vi "encodeArrayVariant.vi"(5 "Cluster To Map? (T)":bool=TRUE, 7 "Compress? (T)":bool=TRUE, 8 "error in":errorcluster, 11 "Variant":variant) -> (0 "error out":errorcluster, 3 "MessagePack":u8[](array[numeric]) format="%.0x")   [LabVIEW 2015, in "MsgPack.lvlib"]
uses:
  MsgPack.lvlib
  encodeArrayInt8.vi
  encodeArrayInt16.vi
  encodeArrayInt32.vi
  encodeArrayInt64.vi
  encodeArrayUInt8.vi
  encodeArrayUInt16.vi
  encodeArrayUInt32.vi
  encodeArrayUInt64.vi
  encodeArrayFloat32.vi
  encodeArrayFloat64.vi
  encodeArrayBoolean.vi
  encodeArrayString.vi
  encodeArrayTimestamp.vi
  encodeBaseType.vi
  encodeInt8.vi
  encodeInt16.vi
  encodeInt32.vi
  encodeInt64.vi
  encodeUInt8.vi
  encodeUInt16.vi
  encodeUInt32.vi
  encodeUInt64.vi
  encodeFloat32.vi
  encodeFloat64.vi
  SubVis/encodeBooleanRaw.vi
  encodeString.vi
  encodeTimestamp.vi
  SubVis/encodeFixedInt.vi
  encodeExt.vi
  <vilib>/ErrorRing/Error Ring.xnode
  <vilib>/Utility/Data Type/NI_Data Type.lvlib
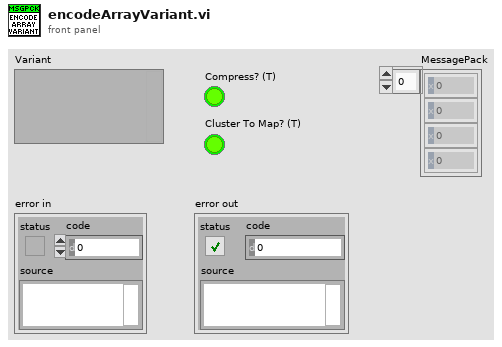
[diagram p1: front panel]
types:
  T1 = typedef "NI_Data Type.lvlib/Data Type.ctl" = enum8{"Invalid Type", "Void", "I8", "I16", "I32", "I64", "U8", "U16", "U32", "U64", "Single Float", "Double Float", "Extended Float", "Single Complex", "Double Complex", "Extended Complex", "Enum U8", "Enum U16", "Enum U32", "Enum U64", "Single Float With Unit", "Double Float With Unit", "Extended Float With Unit", "Single Complex with Unit", "Double Complex with Unit", "Extended Complex with Unit", "Boolean", "String", "Path", "Picture", "Tag", "Array", "Cluster", "Variant", "LV Variant", "Waveform", "Timestamp", "Digital Waveform", "Digital Data", "ExpressData", "Refnum", "External Data", "VI", "Poly VI", "LabVIEW Class Instance", "Fixed Point"}
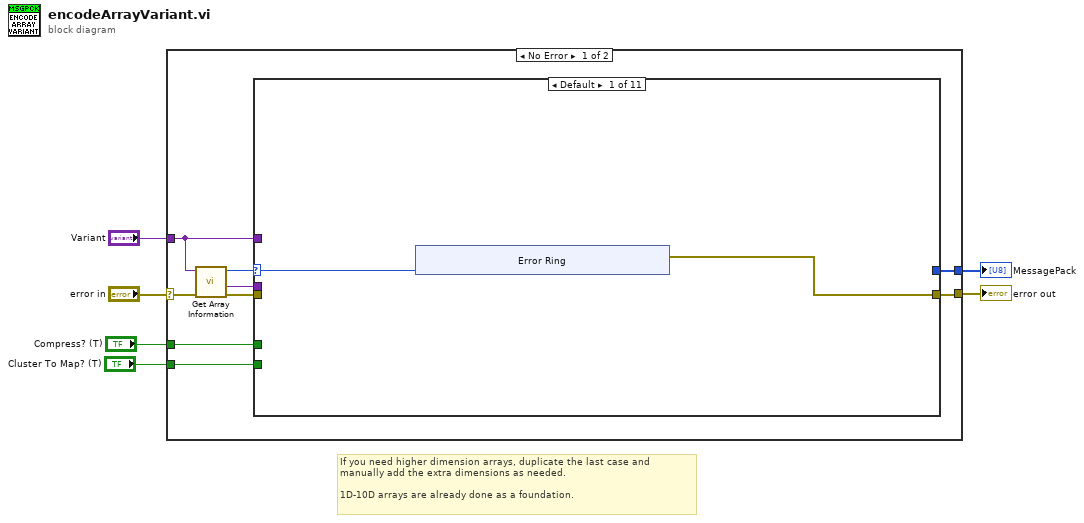
[diagram p0: block diagram]
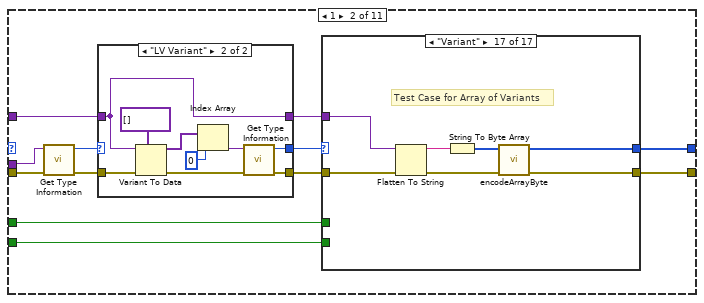
[diagram p2: hidden frame]
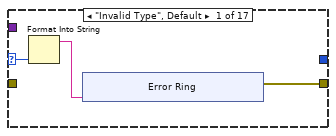
[diagram p4: hidden frame]
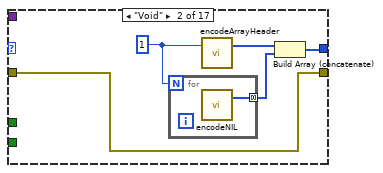
[diagram p5: hidden frame]
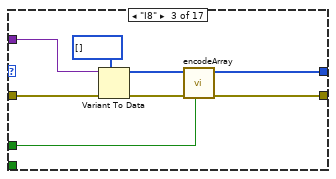
[diagram p6: hidden frame]
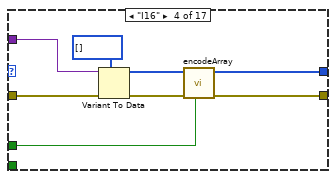
[diagram p7: hidden frame]
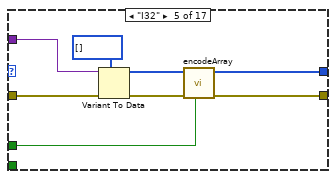
[diagram p8: hidden frame]
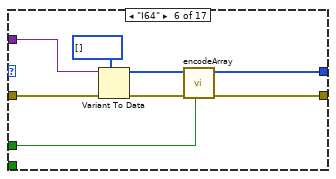
[diagram p9: hidden frame]
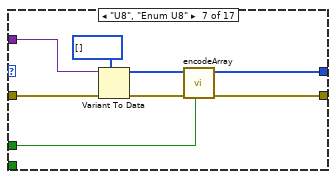
[diagram p10: hidden frame]
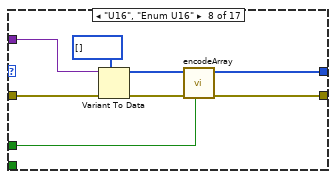
[diagram p11: hidden frame]
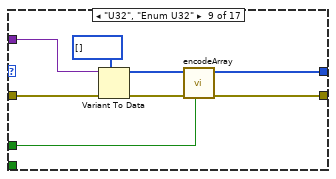
[diagram p12: hidden frame]
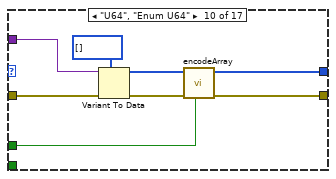
[diagram p13: hidden frame]
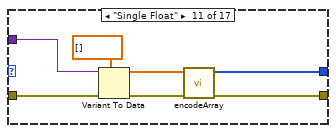
[diagram p14: hidden frame]
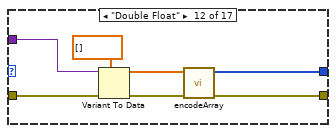
[diagram p15: hidden frame]
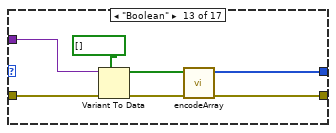
[diagram p16: hidden frame]
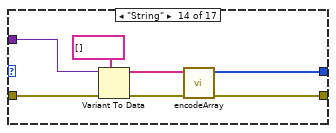
[diagram p17: hidden frame]
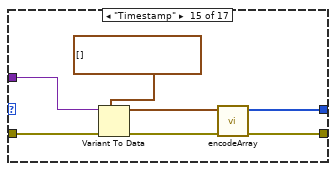
[diagram p18: hidden frame]
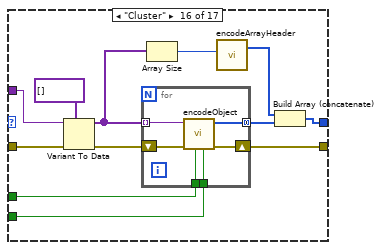
[diagram p19: hidden frame]
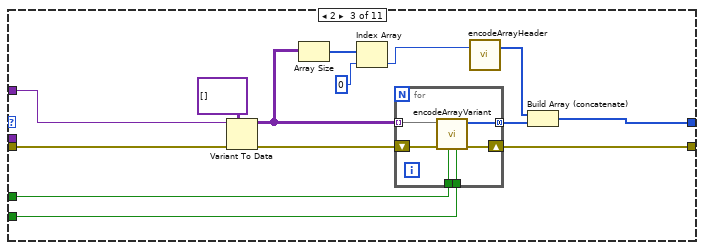
[diagram p20: hidden frame]
diagram:
  # "If you need higher dimension arrays, duplicate the last case and manually add the extra dimensions as needed.\n\n1D-10D arrays are already done as a foundation."
  n1 = case shown="No Error" "error in" {
    selector: "error in" -> [w15 w365]
    tunnel: [w10 _] -> w6
    tunnel: [w9 w365] -> w5
    tunnel: "Variant" -> [w11 _]
    tunnel: "Cluster To Map? (T)" -> [w8 _]
    tunnel: "Compress? (T)" -> [w7 _]
    frame No Error {
      n2 = call <vilib>:"Get Array Information.vi"("error in (no error)"=w15, "Variant"=w11) -> ("error out"=w13:errorcluster, "Array Element Data Type"=w12:variant, "Number of Dimensions"=w14:i32)  [unwired: 6 in, 1 out]
      n3 = case shown="Default" w14 {
        selector: w14 -> [w17 _ _ _ _ _ _ _ _ _ _]
        tunnel: w13 -> [_ w34 w188 w208 w228 w248 w268 w288 w308 w328 w348]
        tunnel: [w16 w32 w198 w218 w238 w258 w278 w298 w318 w338 w358] -> w9
        tunnel: w12 -> [_ w33 _ _ _ _ _ _ _ _ _]
        tunnel: w11 -> [_ w28 w197 w217 w237 w257 w277 w297 w317 w337 w357]
        tunnel: [_ w31 w196 w216 w236 w256 w276 w296 w316 w336 w356] -> w10
        tunnel: w8 -> [_ w30 w195 w215 w235 w255 w275 w295 w315 w335 w355]
        tunnel: w7 -> [_ w29 w194 w214 w234 w254 w274 w294 w314 w334 w354]
        frame Default {
          n4 = xnode "Error Ring"("parameter 0"=w17) -> ("error out"=w16:errorcluster)
        }
        frame 1 {
          n5 = call <vilib>:"Get Type Information.vi"("error in (no error)"=w34, "Variant"=w33) -> ("error out"=w24:errorcluster, "Type"=w26:T1)  [unwired: 5 in, 3 out]
          n6 = case shown="\"LV Variant\"" w26 {
            selector: w26 -> [w37 _]
            tunnel: w28 -> [w36 w38]
            tunnel: [w37 w42] -> w27
            tunnel: [w36 w38] -> w25
            tunnel: w24 -> [w35 w45]
            tunnel: [w35 w40] -> w23
            frame Default {
            }
            frame "LV Variant" {
              n7 = Variant To Data(error in=w45, type=variant[] [] ("Variant Array"), Variant=w38) -> (data=w44:variant[], error out=w41:errorcluster)
              n8 = Index Array(array=w44, index=0) -> (element=w39:variant)
              n9 = call <vilib>:"Get Type Information.vi"("error in (no error)"=w41, "Variant"=w39) -> ("error out"=w40:errorcluster, "Type"=w42:T1)  [unwired: 5 in, 3 out]
            }
          }
          n10 = case shown="\"Variant\"" w27 {
            selector: w27 -> [w48 _ _ _ _ _ _ _ _ _ _ _ _ _ _ _ _]
            tunnel: [w47 w56 w63 w71 w79 w87 w95 w103 w111 w119 w127 w134 w141 w148 w155 w167 w178] -> w32
            tunnel: w23 -> [_ w56 w67 w75 w83 w91 w99 w107 w115 w123 w130 w137 w144 w151 w158 w170 w182]
            tunnel: w25 -> [_ _ w68 w76 w84 w92 w100 w108 w116 w124 w131 w138 w145 w152 w159 w171 w183]
            tunnel: [_ w57 w65 w73 w81 w89 w97 w105 w113 w121 w129 w136 w143 w150 w157 w162 w184] -> w31
            tunnel: w30 -> [_ _ _ _ _ _ _ _ _ _ _ _ _ _ _ w161 _]
            tunnel: w29 -> [_ _ w61 w69 w77 w85 w93 w101 w109 w117 _ _ _ _ _ w160 _]
            frame "Invalid Type", Default {
              n11 = Format Into String(w48) -> (resulting string=w49:string)  [unwired: 3 in, 1 out]
              n12 = xnode "Error Ring"("parameter 0"=w49) -> ("error out"=w47:errorcluster)
            }
            frame "Void" {
              w55 = 1 ("index")
              n13 = for {
                N: w55 -> [_]
                tunnel: [w60] -> w58 mode=concatenating
                n14 = call "encodeNIL.vi"() -> ("MessagePack"=w60:u8[])  [unwired: 3 in]
              }
              n15 = call "encodeArrayHeader.vi"("Number of Elements"=w55) -> ("array header"=w59:u8[])  [unwired: 2 in]
              n16 = Build Array (concatenate)(w59, w58) -> (w57:u8[])
            }
            frame "I8" {
              n17 = Variant To Data(error in=w67, type=i8[] [], Variant=w68) -> (data=w66:i8[], error out=w64:errorcluster)
              n18 = call-poly "encodeArray.vi"("Compress? (T)"=w61, "error in (no error)"=w64, "Int8 Array"=w66) -> ("error out"=w63:errorcluster, "MessagePack"=w65:u8[])  [unwired: 7 in]
            }
            frame "I16" {
              n19 = Variant To Data(error in=w75, type=i16[] [], Variant=w76) -> (data=w74:i16[], error out=w72:errorcluster)
              n20 = call-poly "encodeArray.vi"("Compress? (T)"=w69, "error in (no error)"=w72, "Int16 Array"=w74) -> ("error out"=w71:errorcluster, "MessagePack"=w73:u8[])  [unwired: 7 in]
            }
            frame "I32" {
              n21 = Variant To Data(error in=w83, type=i32[] [], Variant=w84) -> (data=w82:i32[], error out=w80:errorcluster)
              n22 = call-poly "encodeArray.vi"("Compress? (T)"=w77, "error in (no error)"=w80, "Int32 Array"=w82) -> ("error out"=w79:errorcluster, "MessagePack"=w81:u8[])  [unwired: 7 in]
            }
            frame "I64" {
              n23 = Variant To Data(error in=w91, type=i64[] [], Variant=w92) -> (data=w90:i64[], error out=w88:errorcluster)
              n24 = call-poly "encodeArray.vi"("Compress? (T)"=w85, "error in (no error)"=w88, "Int64 Array"=w90) -> ("error out"=w87:errorcluster, "MessagePack"=w89:u8[])  [unwired: 7 in]
            }
            frame "U8", "Enum U8" {
              n25 = Variant To Data(error in=w99, type=u8[] [], Variant=w100) -> (data=w98:u8[], error out=w96:errorcluster)
              n26 = call-poly "encodeArray.vi"("Compress? (T)"=w93, "error in (no error)"=w96, "UInt8 Array"=w98) -> ("error out"=w95:errorcluster, "MessagePack"=w97:u8[])  [unwired: 7 in]
            }
            frame "U16", "Enum U16" {
              n27 = Variant To Data(error in=w107, type=u16[] [], Variant=w108) -> (data=w106:u16[], error out=w104:errorcluster)
              n28 = call-poly "encodeArray.vi"("Compress? (T)"=w101, "error in (no error)"=w104, "UInt16 Array"=w106) -> ("error out"=w103:errorcluster, "MessagePack"=w105:u8[])  [unwired: 7 in]
            }
            frame "U32", "Enum U32" {
              n29 = Variant To Data(error in=w115, type=u32[] [], Variant=w116) -> (data=w114:u32[], error out=w112:errorcluster)
              n30 = call-poly "encodeArray.vi"("Compress? (T)"=w109, "error in (no error)"=w112, "UInt32 Array"=w114) -> ("error out"=w111:errorcluster, "MessagePack"=w113:u8[])  [unwired: 7 in]
            }
            frame "U64", "Enum U64" {
              n31 = Variant To Data(error in=w123, type=u64[] [], Variant=w124) -> (data=w122:u64[], error out=w120:errorcluster)
              n32 = call-poly "encodeArray.vi"("Compress? (T)"=w117, "error in (no error)"=w120, "UInt64 Array"=w122) -> ("error out"=w119:errorcluster, "MessagePack"=w121:u8[])  [unwired: 7 in]
            }
            frame "Single Float" {
              n33 = Variant To Data(error in=w130, type=sgl[] [], Variant=w131) -> (data=w125:sgl[], error out=w128:errorcluster)
              n34 = call-poly "encodeArray.vi"("error in (no error)"=w128, "Single Array"=w125) -> ("error out"=w127:errorcluster, "MessagePack"=w129:u8[])  [unwired: 8 in]
            }
            frame "Double Float" {
              n35 = Variant To Data(error in=w137, type=dbl[] [], Variant=w138) -> (data=w132:dbl[], error out=w135:errorcluster)
              n36 = call-poly "encodeArray.vi"("error in (no error)"=w135, "Double Array"=w132) -> ("error out"=w134:errorcluster, "MessagePack"=w136:u8[])  [unwired: 8 in]
            }
            frame "Boolean" {
              n37 = Variant To Data(error in=w144, type=bool[] [], Variant=w145) -> (data=w139:bool[], error out=w142:errorcluster)
              n38 = call-poly "encodeArray.vi"("error in (no error)"=w142, "Boolean Array"=w139) -> ("error out"=w141:errorcluster, "MessagePack"=w143:u8[])  [unwired: 8 in]
            }
            frame "String" {
              n39 = Variant To Data(error in=w151, type=string[] [], Variant=w152) -> (data=w146:string[], error out=w149:errorcluster)
              n40 = call-poly "encodeArray.vi"("error in (no error)"=w149, "String Array"=w146) -> ("error out"=w148:errorcluster, "MessagePack"=w150:u8[])  [unwired: 8 in]
            }
            frame "Timestamp" {
              n41 = Variant To Data(error in=w158, type=timestamp[] [], Variant=w159) -> (data=w153:timestamp[], error out=w156:errorcluster)
              n42 = call-poly "encodeArray.vi"("error in (no error)"=w156, "Timestamp Array"=w153) -> ("error out"=w155:errorcluster, "MessagePack"=w157:u8[])  [unwired: 8 in]
            }
            frame "Cluster" {
              n43 = Variant To Data(error in=w170, type=variant[] [] ("Variant Array"), Variant=w171) -> (data=w165:variant[], error out=w168:errorcluster)
              n44 = for {
                tunnel: w165 -> [w175] mode=indexing
                shift-right: [w176] -> w167
                shift-left: w168 -> [w177]
                tunnel: [w174] -> w164 mode=concatenating
                tunnel: w161 -> [w173]
                tunnel: w160 -> [w172]
                n45 = call "encodeObject.vi"("Cluster To Map? (T)"=w173, "Compress? (T)"=w172, "error in (no error)"=w177, "Variant"=w175) -> ("error out"=w176:errorcluster, "MessagePack"=w174:u8[])  [unwired: 6 in]
              }
              n46 = Array Size(array=w165) -> (size(s)=w166:i32)
              n47 = call "encodeArrayHeader.vi"("Number of Elements"=w166) -> ("array header"=w163:u8[])  [unwired: 2 in]
              n48 = Build Array (concatenate)(w163, w164) -> (w162:u8[])
            }
            frame "Variant" {
              # "Test Case for Array of Variants"
              n49 = Flatten To String(anything=w183, error in (no error)=w182) -> (data string=w181:string, error out=w179:errorcluster)  [unwired: 2 in, 1 out]
              n50 = String To Byte Array(string=w181) -> (unsigned byte array=w180:u8[])
              n51 = call "encodeArrayByte.vi"("error in (no error)"=w179, "Byte Array"=w180) -> ("error out"=w178:errorcluster, "MessagePack"=w184:u8[])  [unwired: 8 in]
            }
          }
        }
        frame 2 {
          n52 = Variant To Data(error in=w188, type=variant[][] [] ("Variant Array"), Variant=w197) -> (data=w191:variant[][], error out=w192:errorcluster)
          n53 = Array Size(array=w191) -> (size(s)=w187:i32[])
          n54 = Index Array(array=w187, index=0) -> (element=w186:i32)
          n55 = for {
            tunnel: w191 -> [w201] mode=indexing
            shift-right: [w199] -> w198
            shift-left: w192 -> [w200]
            tunnel: [w204] -> w190 mode=concatenating
            tunnel: w195 -> [w203]
            tunnel: w194 -> [w202]
            n56 = call "encodeArrayVariant.vi"("Cluster To Map? (T)"=w203, "Compress? (T)"=w202, "error in"=w200, "Variant"=w201) -> ("error out"=w199:errorcluster, "MessagePack"=w204:u8[])  [unwired: 6 in]
          }
          n57 = call "encodeArrayHeader.vi"("Number of Elements"=w186) -> ("array header"=w189:u8[])  [unwired: 2 in]
          n58 = Build Array (concatenate)(w189, w190) -> (w196:u8[])
        }
        frame 3 {
          n59 = Variant To Data(error in=w208, type=variant[][][] [] ("Variant Array"), Variant=w217) -> (data=w211:variant[][][], error out=w212:errorcluster)
          n60 = Array Size(array=w211) -> (size(s)=w207:i32[])
          n61 = Index Array(array=w207, index=0) -> (element=w206:i32)
          n62 = for {
            tunnel: w211 -> [w221] mode=indexing
            shift-right: [w219] -> w218
            shift-left: w212 -> [w220]
            tunnel: [w224] -> w210 mode=concatenating
            tunnel: w215 -> [w223]
            tunnel: w214 -> [w222]
            n63 = call "encodeArrayVariant.vi"("Cluster To Map? (T)"=w223, "Compress? (T)"=w222, "error in"=w220, "Variant"=w221) -> ("error out"=w219:errorcluster, "MessagePack"=w224:u8[])  [unwired: 6 in]
          }
          n64 = call "encodeArrayHeader.vi"("Number of Elements"=w206) -> ("array header"=w209:u8[])  [unwired: 2 in]
          n65 = Build Array (concatenate)(w209, w210) -> (w216:u8[])
        }
        frame 4 {
          n66 = Variant To Data(error in=w228, type=variant[][][][] [] ("Variant Array"), Variant=w237) -> (data=w231:variant[][][][], error out=w232:errorcluster)
          n67 = Array Size(array=w231) -> (size(s)=w227:i32[])
          n68 = Index Array(array=w227, index=0) -> (element=w226:i32)
          n69 = for {
            tunnel: w231 -> [w241] mode=indexing
            shift-right: [w239] -> w238
            shift-left: w232 -> [w240]
            tunnel: [w244] -> w230 mode=concatenating
            tunnel: w235 -> [w243]
            tunnel: w234 -> [w242]
            n70 = call "encodeArrayVariant.vi"("Cluster To Map? (T)"=w243, "Compress? (T)"=w242, "error in"=w240, "Variant"=w241) -> ("error out"=w239:errorcluster, "MessagePack"=w244:u8[])  [unwired: 6 in]
          }
          n71 = call "encodeArrayHeader.vi"("Number of Elements"=w226) -> ("array header"=w229:u8[])  [unwired: 2 in]
          n72 = Build Array (concatenate)(w229, w230) -> (w236:u8[])
        }
        frame 5 {
          n73 = Variant To Data(error in=w248, type=variant[][][][][] [] ("Variant Array"), Variant=w257) -> (data=w251:variant[][][][][], error out=w252:errorcluster)
          n74 = Array Size(array=w251) -> (size(s)=w247:i32[])
          n75 = Index Array(array=w247, index=0) -> (element=w246:i32)
          n76 = for {
            tunnel: w251 -> [w261] mode=indexing
            shift-right: [w259] -> w258
            shift-left: w252 -> [w260]
            tunnel: [w264] -> w250 mode=concatenating
            tunnel: w255 -> [w263]
            tunnel: w254 -> [w262]
            n77 = call "encodeArrayVariant.vi"("Cluster To Map? (T)"=w263, "Compress? (T)"=w262, "error in"=w260, "Variant"=w261) -> ("error out"=w259:errorcluster, "MessagePack"=w264:u8[])  [unwired: 6 in]
          }
          n78 = call "encodeArrayHeader.vi"("Number of Elements"=w246) -> ("array header"=w249:u8[])  [unwired: 2 in]
          n79 = Build Array (concatenate)(w249, w250) -> (w256:u8[])
        }
        frame 6 {
          n80 = Variant To Data(error in=w268, type=variant[][][][][][] [] ("Variant Array"), Variant=w277) -> (data=w271:variant[][][][][][], error out=w272:errorcluster)
          n81 = Array Size(array=w271) -> (size(s)=w267:i32[])
          n82 = Index Array(array=w267, index=0) -> (element=w266:i32)
          n83 = for {
            tunnel: w271 -> [w281] mode=indexing
            shift-right: [w279] -> w278
            shift-left: w272 -> [w280]
            tunnel: [w284] -> w270 mode=concatenating
            tunnel: w275 -> [w283]
            tunnel: w274 -> [w282]
            n84 = call "encodeArrayVariant.vi"("Cluster To Map? (T)"=w283, "Compress? (T)"=w282, "error in"=w280, "Variant"=w281) -> ("error out"=w279:errorcluster, "MessagePack"=w284:u8[])  [unwired: 6 in]
          }
          n85 = call "encodeArrayHeader.vi"("Number of Elements"=w266) -> ("array header"=w269:u8[])  [unwired: 2 in]
          n86 = Build Array (concatenate)(w269, w270) -> (w276:u8[])
        }
        frame 7 {
          n87 = Variant To Data(error in=w288, type=variant[][][][][][][] [] ("Variant Array"), Variant=w297) -> (data=w291:variant[][][][][][][], error out=w292:errorcluster)
          n88 = Array Size(array=w291) -> (size(s)=w287:i32[])
          n89 = Index Array(array=w287, index=0) -> (element=w286:i32)
          n90 = for {
            tunnel: w291 -> [w301] mode=indexing
            shift-right: [w299] -> w298
            shift-left: w292 -> [w300]
            tunnel: [w304] -> w290 mode=concatenating
            tunnel: w295 -> [w303]
            tunnel: w294 -> [w302]
            n91 = call "encodeArrayVariant.vi"("Cluster To Map? (T)"=w303, "Compress? (T)"=w302, "error in"=w300, "Variant"=w301) -> ("error out"=w299:errorcluster, "MessagePack"=w304:u8[])  [unwired: 6 in]
          }
          n92 = call "encodeArrayHeader.vi"("Number of Elements"=w286) -> ("array header"=w289:u8[])  [unwired: 2 in]
          n93 = Build Array (concatenate)(w289, w290) -> (w296:u8[])
        }
        frame 8 {
          n94 = Variant To Data(error in=w308, type=variant[][][][][][][][] [] ("Variant Array"), Variant=w317) -> (data=w311:variant[][][][][][][][], error out=w312:errorcluster)
          n95 = Array Size(array=w311) -> (size(s)=w307:i32[])
          n96 = Index Array(array=w307, index=0) -> (element=w306:i32)
          n97 = for {
            tunnel: w311 -> [w321] mode=indexing
            shift-right: [w319] -> w318
            shift-left: w312 -> [w320]
            tunnel: [w324] -> w310 mode=concatenating
            tunnel: w315 -> [w323]
            tunnel: w314 -> [w322]
            n98 = call "encodeArrayVariant.vi"("Cluster To Map? (T)"=w323, "Compress? (T)"=w322, "error in"=w320, "Variant"=w321) -> ("error out"=w319:errorcluster, "MessagePack"=w324:u8[])  [unwired: 6 in]
          }
          n99 = call "encodeArrayHeader.vi"("Number of Elements"=w306) -> ("array header"=w309:u8[])  [unwired: 2 in]
          n100 = Build Array (concatenate)(w309, w310) -> (w316:u8[])
        }
        frame 9 {
          n101 = Variant To Data(error in=w328, type=variant[][][][][][][][][] [] ("Variant Array"), Variant=w337) -> (data=w331:variant[][][][][][][][][], error out=w332:errorcluster)
          n102 = Array Size(array=w331) -> (size(s)=w327:i32[])
          n103 = Index Array(array=w327, index=0) -> (element=w326:i32)
          n104 = for {
            tunnel: w331 -> [w341] mode=indexing
            shift-right: [w339] -> w338
            shift-left: w332 -> [w340]
            tunnel: [w344] -> w330 mode=concatenating
            tunnel: w335 -> [w343]
            tunnel: w334 -> [w342]
            n105 = call "encodeArrayVariant.vi"("Cluster To Map? (T)"=w343, "Compress? (T)"=w342, "error in"=w340, "Variant"=w341) -> ("error out"=w339:errorcluster, "MessagePack"=w344:u8[])  [unwired: 6 in]
          }
          n106 = call "encodeArrayHeader.vi"("Number of Elements"=w326) -> ("array header"=w329:u8[])  [unwired: 2 in]
          n107 = Build Array (concatenate)(w329, w330) -> (w336:u8[])
        }
        frame 10 {
          n108 = Variant To Data(error in=w348, type=variant[][][][][][][][][][] [] ("Variant Array"), Variant=w357) -> (data=w351:variant[][][][][][][][][][], error out=w352:errorcluster)
          n109 = Array Size(array=w351) -> (size(s)=w347:i32[])
          n110 = Index Array(array=w347, index=0) -> (element=w346:i32)
          n111 = for {
            tunnel: w351 -> [w361] mode=indexing
            shift-right: [w359] -> w358
            shift-left: w352 -> [w360]
            tunnel: [w364] -> w350 mode=concatenating
            tunnel: w355 -> [w363]
            tunnel: w354 -> [w362]
            n112 = call "encodeArrayVariant.vi"("Cluster To Map? (T)"=w363, "Compress? (T)"=w362, "error in"=w360, "Variant"=w361) -> ("error out"=w359:errorcluster, "MessagePack"=w364:u8[])  [unwired: 6 in]
          }
          n113 = call "encodeArrayHeader.vi"("Number of Elements"=w346) -> ("array header"=w349:u8[])  [unwired: 2 in]
          n114 = Build Array (concatenate)(w349, w350) -> (w356:u8[])
        }
      }
    }
    frame Error {
    }
  }
  "MessagePack" <- w6
  "error out" <- w5
